vi "test-trajectory-transform.vi"() -> ()   [LabVIEW 2019]
uses:
  <vilib>/Rock Robotics/WPI/ThirdParty/JAS_Junk/TrajLib/TRAJECTORY.ctl
  <vilib>/Rock Robotics/WPI/ThirdParty/JAS_Junk/TrajLib/TRAJ_STATE.ctl
  <vilib>/Rock Robotics/WPI/ThirdParty/JAS_Junk/TrajLib/POSE2D.ctl
  <vilib>/Rock Robotics/WPI/ThirdParty/JAS_Junk/TrajLib/TRANSLATION2D.ctl
  <vilib>/Rock Robotics/WPI/ThirdParty/JAS_Junk/TrajLib/ROTATION2D.ctl
  <vilib>/Rock Robotics/WPI/ThirdParty/JAS_Junk/TrajLib/Trajectory_Library.lvlib
panel:
  out "XY Graph 2":cluster{dbl[], dbl[]}[](graph)
  out "outputTRAJECTORY 2":T1 {"States"."POSE"."ROTATION"."SIN" format="%13.4f"; "States"."POSE"."ROTATION"."COS" format="%13.4f"; "States"."POSE"."ROTATION"."VALUE" format="%13.4f"; "States"."POSE"."TRANSLATION"."Y" format="%14.3f"; "States"."POSE"."TRANSLATION"."X" format="%14.3f"; "TotalTImeSecs" format="%20.3f"}
  out "TRAJECTORY 2":T1 {"States"."POSE"."ROTATION"."SIN" format="%13.4f"; "States"."POSE"."ROTATION"."COS" format="%13.4f"; "States"."POSE"."ROTATION"."VALUE" format="%13.4f"; "States"."POSE"."TRANSLATION"."Y" format="%14.3f"; "States"."POSE"."TRANSLATION"."X" format="%14.3f"; "TotalTImeSecs" format="%20.3f"}
  out "XY Graph":cluster{dbl[], dbl[]}[](graph)
  out "outputTRAJECTORY":T1 {"States"."POSE"."ROTATION"."SIN" format="%13.4f"; "States"."POSE"."ROTATION"."COS" format="%13.4f"; "States"."POSE"."ROTATION"."VALUE" format="%13.4f"; "States"."POSE"."TRANSLATION"."Y" format="%14.3f"; "States"."POSE"."TRANSLATION"."X" format="%14.3f"; "TotalTImeSecs" format="%20.3f"}
  out "TRAJECTORY":T1 {"States"."POSE"."ROTATION"."SIN" format="%13.4f"; "States"."POSE"."ROTATION"."COS" format="%13.4f"; "States"."POSE"."ROTATION"."VALUE" format="%13.4f"; "States"."POSE"."TRANSLATION"."Y" format="%14.3f"; "States"."POSE"."TRANSLATION"."X" format="%14.3f"; "TotalTImeSecs" format="%20.3f"}
  # "Trajectory Transform"
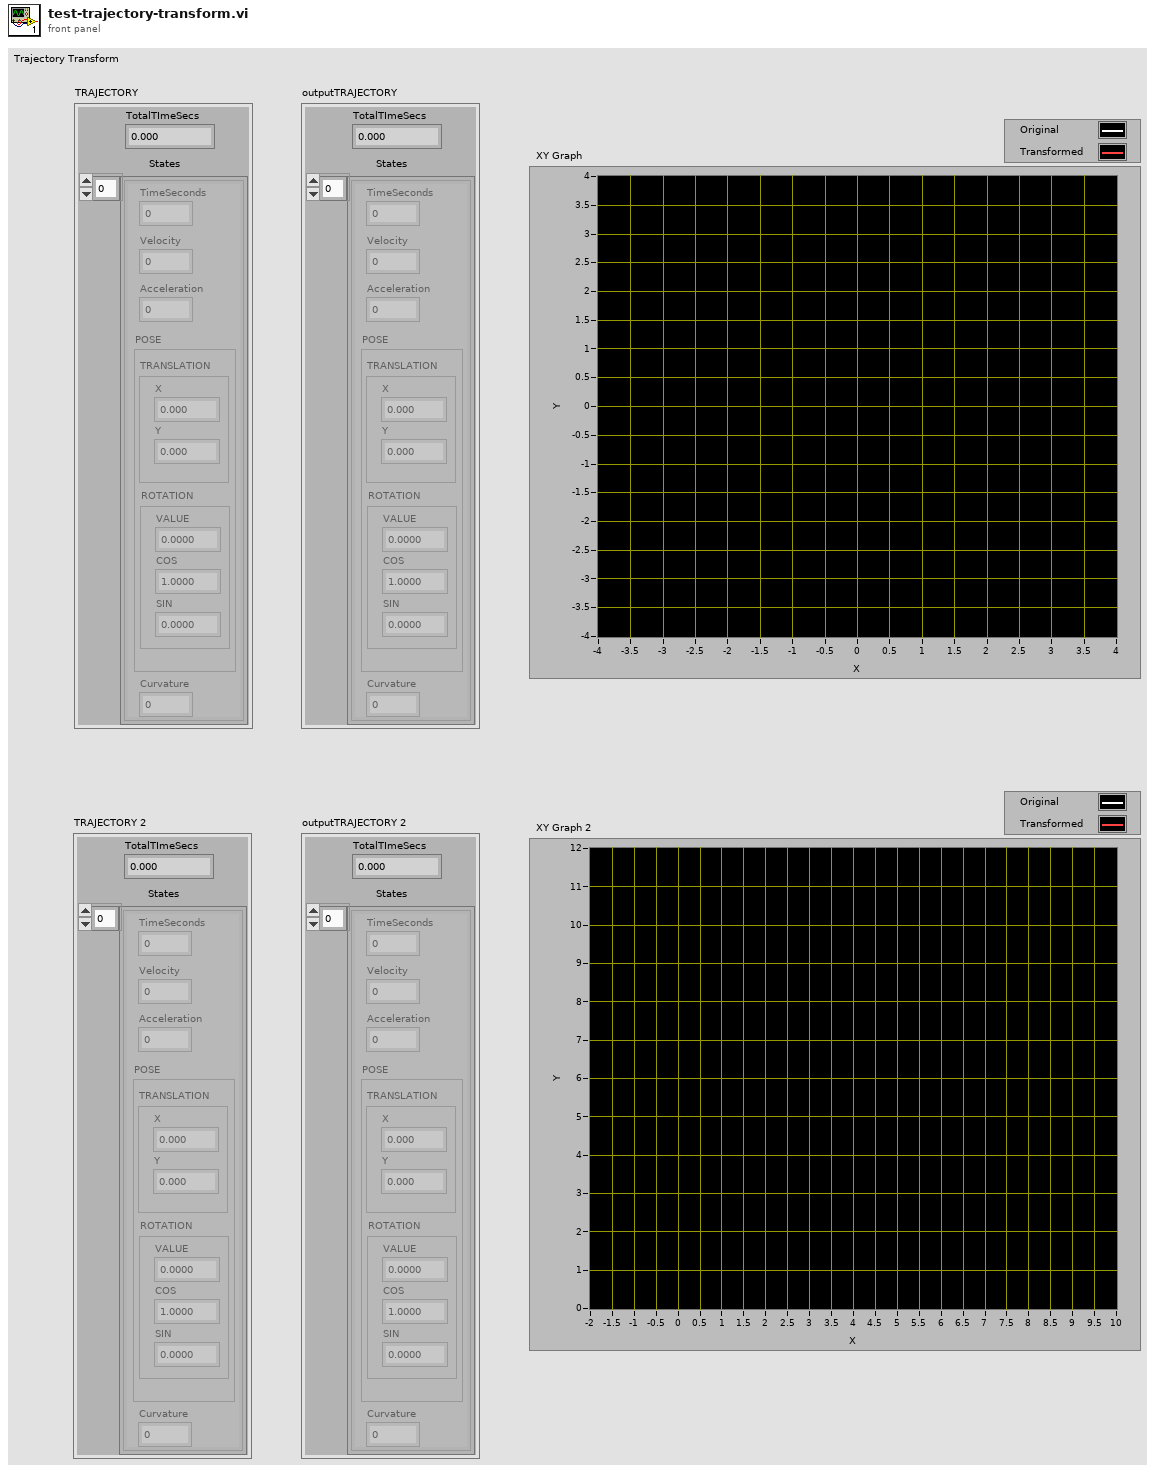
[diagram p1: front panel]
types:
  T1 = typedef "Trajectory_Library.lvlib/TRAJECTORY.ctl" = cluster{"TotalTImeSecs":dbl, "States":T2[]}
  T2 = typedef "Trajectory_Library.lvlib/TRAJ_STATE.ctl" = cluster{"TimeSeconds":dbl, "Velocity":dbl, "Acceleration":dbl, "POSE":T3, "Curvature":dbl}
  T3 = typedef "Trajectory_Library.lvlib/POSE2D.ctl" = cluster{"TRANSLATION":T4, "ROTATION":T5}
  T4 = typedef "Trajectory_Library.lvlib/TRANSLATION2D.ctl" = cluster{"X":dbl, "Y":dbl}
  T5 = typedef "Trajectory_Library.lvlib/ROTATION2D.ctl" = cluster{"VALUE":dbl, "COS":dbl, "SIN":dbl}
  T6 = typedef "Trajectory_Library.lvlib/TRAJ_CONFIG.ctl" = cluster{"MaxVelocity":dbl, "Max Acceleration":dbl, "StartVelocity":dbl, "End Velocity":dbl, "Reversed":bool, "DiffDrKineConstntDefined":bool, "CentAcellConstntDefined":bool, "DiffDrVoltConstntDefined":bool, "DIFF_DRIVE_KINE_CONSTRAINT":T7, "CENTRIPETAL_ACCEL_CONSTRAINT":T9, "SwerveDrKineConstntDefined":bool, "SWERVE_DRIVE_KINE_CONSTRAINT":T10, "DIFF_DRIVE_VOLTAGE_CONSTRAINT":T13, "MECANUM_DRIVE_KINE_CONSTRAINT":T15, "MecanumDrKineConstntDefined":bool}
  T7 = typedef "Trajectory_Library.lvlib/TRAJ_CONSTRAINT_DIIF_DRIVE_KINEMATICS.ctl" = cluster{"Max Speed (M/S)":dbl, "DIFF_DRIVE_KINEMATICS":T8}
  T8 = typedef "Trajectory_Library.lvlib/DIFF_DRIVE_KINEMATICS.ctl" = cluster{"TrackWidth_Meters":dbl}
  T9 = typedef "Trajectory_Library.lvlib/TRAJ_CONSTRAINT_CENTRIPETAL_ACCEL.ctl" = cluster{"Max Cent Accel":dbl}
  T10 = typedef "Trajectory_Library.lvlib/TRAJ_CONSTRAINT_SWERVE_DRIVE_KINEMATICS.ctl" = cluster{"Max Speed (M/S)":dbl, "SwerveKinematics":T11}
  T11 = typedef "Trajectory_Library.lvlib/SWERVE_DRIVE_KINEMATICS.ctl" = cluster{"NumModules":i32, "InverseKinematics":T12, "ForwardKinematics":T12, "Modules":T4[], "PrevCoR":T4}
  T12 = typedef "NI_Matrix.lvlib/RealMatrix.ctl" = dbl[][]
  T13 = typedef "Trajectory_Library.lvlib/TRAJ_CONSTRAINT_DIIF_DRIVE_VOLTAGE.ctl" = cluster{"Max Voltage":dbl, "DIFF_DRIVE_KINEMATICS":T8, "SIMPLE_MOTOR_FF":T14}
  T14 = typedef "Trajectory_Library.lvlib/SIMPLE_MOTOR_FF.ctl" = cluster{"Ks":dbl, "Kv":dbl, "Ka":dbl}
  T15 = typedef "Trajectory_Library.lvlib/TRAJ_CONSTRAINT_MECA_DRIVE_KINEMATICS.ctl" = cluster{"Max Speed (M/S)":dbl, "MECA_DRIVE_KINEMATICS":T16}
  T16 = typedef "Trajectory_Library.lvlib/MECA_DRIVE_KINEMATICS.ctl" = cluster{"FrontLeft":T4, "FrontRight":T4, "RearLeft":T4, "RearRight":T4, "InverseKinematics":T12, "ForwardKinematics":T12, "PrevCoR":T4}
  T17 = typedef "Trajectory_Library.lvlib/TRANSFORM2D.ctl" = cluster{"TRANSLATION":T4, "ROTATION":T5}
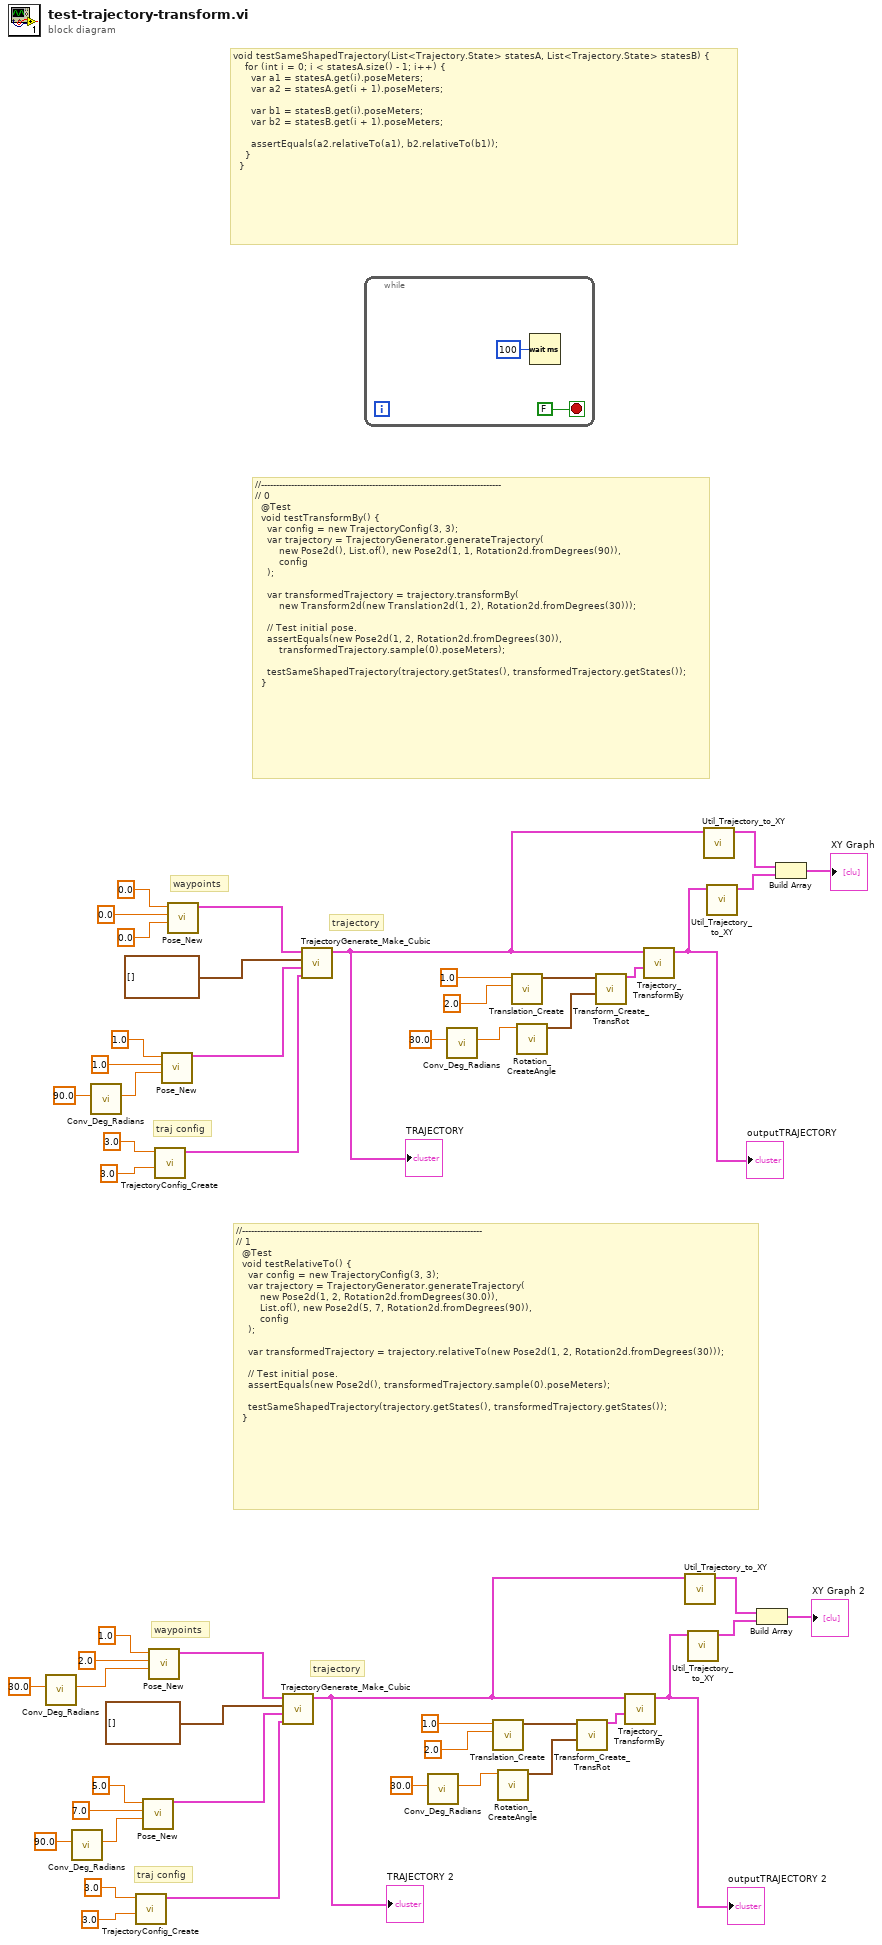
[diagram p0: block diagram]
diagram:
  # "void testSameShapedTrajectory(List<Trajectory.State> statesA, List<Trajectory.State> statesB) {\n    for (int i = 0; i < statesA.size() - 1; i++) {\n      var a1 = statesA.get(i).poseMeters;\n      var a2 = statesA.get(i + 1).poseMeters;\n\n      var b1 = statesB.get(i).poseMeters;\n      var b2 = statesB.get(i + 1).poseMeters;\n\n      assertEquals(a2.relativeTo(a1), b2.relativeTo(b1));\n    }\n  }"
  # "traj config"
  # "trajectory"
  # "waypoints"
  # "//--------------------------------------------------------------------------------\n// 1\n  @Test\n  void testRelativeTo() {\n    var config = new TrajectoryConfig(3, 3);\n    var trajectory = TrajectoryGenerator.generateTrajectory(\n        new Pose2d(1, 2, Rotation2d.fromDegrees(30.0)),\n        List.of(), new Pose2d(5, 7, Rotation2d.fromDegrees(90)),\n        config\n    );\n\n    var transformedTrajectory = trajectory.relativeTo(new Pose2d(1, 2, Rotation2d.fromDegrees(30)));\n\n    // Test initial pose.\n    assertEquals(new Pose2d(), transformedTrajectory.sample(0).poseMeters);\n\n    testSameShapedTrajectory(trajectory.getStates(), transformedTrajectory.getStates());\n  }"
  # "traj config"
  # "trajectory"
  # "waypoints"
  # "//--------------------------------------------------------------------------------\n// 0\n  @Test\n  void testTransformBy() {\n    var config = new TrajectoryConfig(3, 3);\n    var trajectory = TrajectoryGenerator.generateTrajectory(\n        new Pose2d(), List.of(), new Pose2d(1, 1, Rotation2d.fromDegrees(90)),\n        config\n    );\n\n    var transformedTrajectory = trajectory.transformBy(\n        new Transform2d(new Translation2d(1, 2), Rotation2d.fromDegrees(30)));\n\n    // Test initial pose.\n    assertEquals(new Pose2d(1, 2, Rotation2d.fromDegrees(30)),\n        transformedTrajectory.sample(0).poseMeters);\n\n    testSameShapedTrajectory(trajectory.getStates(), transformedTrajectory.getStates());\n  }"
  n1 = call <vilib>:"Conv_Deg_Radians.vi"("Degress"=30.0 ("Heading")) -> ("Radians"=w1:dbl)  [unwired: 10 in]
  n2 = call <vilib>:"Conv_Deg_Radians.vi"("Degress"=90.0 ("Heading")) -> ("Radians"=w20:dbl)  [unwired: 10 in]
  n3 = call <vilib>:"Conv_Deg_Radians.vi"("Degress"=90.0 ("Heading")) -> ("Radians"=w44:dbl)  [unwired: 10 in]
  n4 = call <vilib>:"TrajectoryConfig_Create.vi"("MaxAcceleration"=3.0, "MaxVelocity"=3.0) -> ("TRAJECTORY_CONFIG"=w18:T6)  [unwired: 9 in]
  n5 = call <vilib>:"Pose_New.vi"("Heading"=w20, "Y"=7.0, "X"=5.0) -> ("out POSe"=w17:T3)  [unwired: 8 in]
  n6 = call <vilib>:"Pose_New.vi"("Heading"=w1, "Y"=2.0, "X"=1.0) -> ("out POSe"=w16:T3)  [unwired: 8 in]
  n7 = call <vilib>:"TrajectoryConfig_Create.vi"("MaxAcceleration"=3.0, "MaxVelocity"=3.0) -> ("TRAJECTORY_CONFIG"=w42:T6)  [unwired: 9 in]
  n8 = call <vilib>:"Pose_New.vi"("Heading"=w44, "Y"=1.0, "X"=1.0) -> ("out POSe"=w41:T3)  [unwired: 8 in]
  n9 = call <vilib>:"Pose_New.vi"("Heading"=0.0, "Y"=0.0, "X"=0.0) -> ("out POSe"=w40:T3)  [unwired: 8 in]
  n10 = call <vilib>:"TrajectoryGenerate_Make_Cubic.vi"("traj_config"=w18, "Enging POSE"=w17, "Interior WAYPOINTS"=T4[] [], "Starting POSE"=w16) -> ("TRAJECTORY"=w6:T1)  [unwired: 6 in, 1 out]
  "TRAJECTORY 2" <- w6
  n11 = call <vilib>:"TrajectoryGenerate_Make_Cubic.vi"("traj_config"=w42, "Enging POSE"=w41, "Interior WAYPOINTS"=T4[] [], "Starting POSE"=w40) -> ("TRAJECTORY"=w30:T1)  [unwired: 6 in, 1 out]
  "TRAJECTORY" <- w30
  n12 = while {
    stop <- FALSE stop-if-true
    n13 = Wait (ms)(milliseconds to wait=u32 100) -> ()  [unwired: 1 out]
  }
  n14 = call <vilib>:"Conv_Deg_Radians.vi"("Degress"=30.0 ("Heading")) -> ("Radians"=w10:dbl)  [unwired: 10 in]
  n15 = call <vilib>:"Conv_Deg_Radians.vi"("Degress"=30.0 ("Heading")) -> ("Radians"=w34:dbl)  [unwired: 10 in]
  n16 = call <vilib>:"Translation_Create.vi"("Y"=2.0, "X"=1.0) -> ("TRANSLATION"=w14:T4)  [unwired: 9 in]
  n17 = call <vilib>:"Rotation_CreateAngle.vi"("Angle"=w10) -> ("ROTATION"=w13:T5)  [unwired: 10 in]
  n18 = call <vilib>:"Translation_Create.vi"("Y"=2.0, "X"=1.0) -> ("TRANSLATION"=w38:T4)  [unwired: 9 in]
  n19 = call <vilib>:"Rotation_CreateAngle.vi"("Angle"=w34) -> ("ROTATION"=w37:T5)  [unwired: 10 in]
  n20 = call <vilib>:"Transform_Create_TransRot.vi"("ROTATION"=w13, "TRANSLATION"=w14) -> ("TRANSFORM"=w12:T17)  [unwired: 9 in]
  n21 = call <vilib>:"Transform_Create_TransRot.vi"("ROTATION"=w37, "TRANSLATION"=w38) -> ("TRANSFORM"=w36:T17)  [unwired: 9 in]
  n22 = call <vilib>:"Trajectory_TransformBy.vi"("TRANSFORM"=w12, "InputTRAJECTORY"=w6) -> ("outputTRAJECTORY"=w7:T1)  [unwired: 9 in]
  "outputTRAJECTORY 2" <- w7
  n23 = call <vilib>:"Trajectory_TransformBy.vi"("TRANSFORM"=w36, "InputTRAJECTORY"=w30) -> ("outputTRAJECTORY"=w31:T1)  [unwired: 9 in]
  "outputTRAJECTORY" <- w31
  n24 = call <vilib>:"Util_Trajectory_to_XY.vi"("TRAJECTORY"=w6) -> ("outArrayXY"=w4:cluster{dbl[], dbl[]})  [unwired: 10 in]
  n25 = call <vilib>:"Util_Trajectory_to_XY.vi"("TRAJECTORY"=w7) -> ("outArrayXY"=w3:cluster{dbl[], dbl[]})  [unwired: 10 in]
  n26 = call <vilib>:"Util_Trajectory_to_XY.vi"("TRAJECTORY"=w30) -> ("outArrayXY"=w28:cluster{dbl[], dbl[]})  [unwired: 10 in]
  n27 = call <vilib>:"Util_Trajectory_to_XY.vi"("TRAJECTORY"=w31) -> ("outArrayXY"=w27:cluster{dbl[], dbl[]})  [unwired: 10 in]
  n28 = Build Array(w4, w3) -> (→"XY Graph 2":cluster{dbl[], dbl[]}[])
  n29 = Build Array(w28, w27) -> (→"XY Graph":cluster{dbl[], dbl[]}[])
